vi "RSZVB Query Trace Add S-Parameter Group.vi"(8 "error in (no error)":errorcluster {"code" format="%.0x"}, 10 "Channel (1)":i32=1, 11 "VISA session":refnum<visa-resource-name>) -> (0 "error out":errorcluster {"code" format="%.0x"}, 1 "Logical Port Number":i32[](array[numeric]), 3 "dup VISA session":refnum<visa-resource-name>)   [LabVIEW 2011]
doc: "This VI returns a group of logical ports (S-parameter group). \n\nRemote-control command(s):\nCALCulate<Ch>:PARameter:DEFine:SGRoup?"
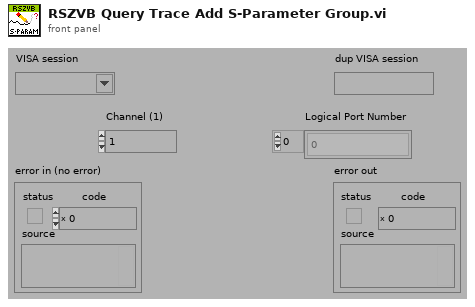
[diagram p1: front panel]
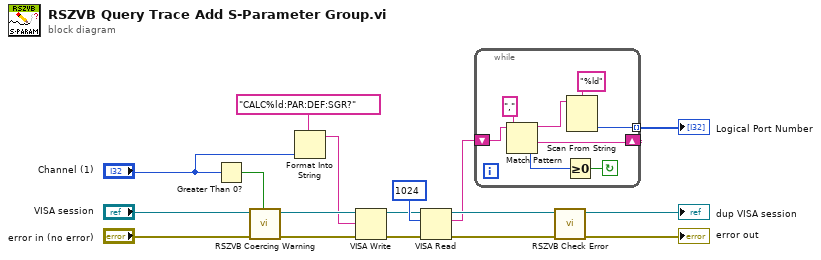
[diagram p0: block diagram]
diagram:
  n1 = Greater Than 0?(x="Channel (1)") -> (x > 0?=w6:bool)
  n2 = call "RSZVB Coercing Warning.vi"("In Range?"=w6, "error in (no error)"="error in (no error)", "VISA session"="VISA session") -> ("error out"=w16:errorcluster, "dup VISA session"=w17:refnum<visa-resource-name>)  [unwired: 7 in]
  n3 = Format Into String(format string="CALC%ld:PAR:DEF:SGR?", "Channel (1)") -> (resulting string=w9:string)  [unwired: 2 in, 1 out]
  n4 = VISA Write(VISA resource name=w17, write buffer=w9, error in (no error)=w16) -> (VISA resource name out=w11:refnum<visa-resource-name>, error out=w12:errorcluster)  [unwired: 1 out]
  n5 = VISA Read(VISA resource name=w11, byte count=u32 1024 ("byte count (0)"), error in (no error)=w12) -> (VISA resource name out=w15:refnum<visa-resource-name>, read buffer=w8:string, error out=w14:errorcluster)  [unwired: 1 out]
  n6 = while {
    shift-left: w8 -> [w23]
    shift-right: [w22] -> _
    tunnel: [w18] -> w1 mode=indexing
    stop <- w20 continue-if-true
    n7 = Match Pattern(string=w23, regular expression=",") -> (before substring=w21:string, after substring=w22:string, offset past match=w19:i32)  [unwired: 1 in, 1 out]
    n8 = Greater Or Equal To 0?(x=w19) -> (x >= 0?=w20:bool)
    n9 = Scan From String(format string="%ld", input string=w21) -> (output 1=w18:i32)  [unwired: 3 in, 3 out]
  }
  "Logical Port Number" <- w1
  n10 = call "RSZVB Check Error.vi"("error in (no error)"=w14, "VISA session"=w15) -> ("error out"=→"error out":errorcluster, "dup VISA session"=→"dup VISA session":refnum<visa-resource-name>)  [unwired: 8 in]
